vi "Launcher.vi"   [LabVIEW 2020]
uses:
  ParentActor/ParentActor.lvclass
  C:/Program Files (x86)/National Instruments/LabVIEW 2020/vi.lib/ActorFramework/Actor/Actor.lvclass
  <vilib>/ActorFramework/Actor/Actor.lvclass
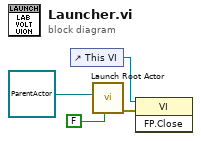
[diagram p0: block diagram]
diagram:
  n1 = control-ref of="This VI"() -> (w3:refnum<vi>)
  n2 = call <vilib>:"Launch Root Actor.vi"("Open Actor Core front panel? (F)"=FALSE, "Actor"=refnum<class "ParentActor.lvclass"> refnum ("ParentActor.lvclass")) -> ("error out"=w1:errorcluster)  [unwired: 8 in, 1 out]
  n3 = invoke class="VI" method="FP.Close"(reference=w3, error in=w1) -> ()  [unwired: 1 in, 3 out]
